vi "Cleanup.vi"(8 "error in (no error)":errorcluster, 11 "Message Maker in":refnum<class "Message Maker.lvclass">) -> (0 "error out":errorcluster)   [LabVIEW 2023, in "Message Maker.lvclass"]
doc: "Closes opened references\n\nAuthor: Derek Trepanier\nCopyright: MGI 2015"
uses:
  Message Maker.lvclass
  Message Maker.lvclass/Message Maker.ctl
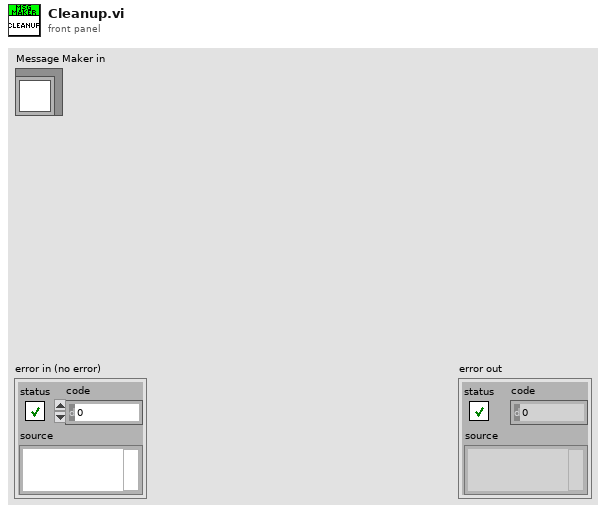
[diagram p1: front panel]
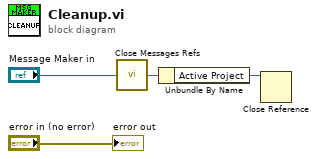
[diagram p0: block diagram]
diagram:
  n1 = call "Close Messages Refs.vi"("Message Maker in"="Message Maker in") -> ("Message Maker out"=w1:refnum<class "Message Maker.lvclass">)
  n2 = Unbundle By Name(w1) -> ("Active Project"=w3:refnum<vi>)
  n3 = Close Reference(reference=w3) -> ()  [unwired: 1 in, 1 out]
  "error out" <- "error in (no error)"
